vi "Version_2.0_Single_Column_Code.vi"() -> ()   [LabVIEW 2020] (continued)
                                n7327 = call "ProcessCompletionWaiter (SubVI).vi"("VISA Refnum in"=w7772) -> ()  [unwired: 11 in]
                                n7328 = local write "Start the Process"(FALSE ("Start the Process")) -> ()
                              }
                            }
                          }
                          frame #13 {
                            # "Clean the tubing with Sample"
                            n7329 = local read "N-S"() -> (w7774:i32)
                            n7330 = for {
                              N: w7774 -> [_]
                              n7331 = stacked-sequence {
                                frame #0 {
                                n7332 = local read "VISA Refnum in\nfor Pump"() -> (w7777:refnum<visa-resource-name>)
                                n7333 = local read "Port for \nSample"() -> (w7776:string)
                                n7334 = call "PortChanger (SubVI).vi"("Port Number"=w7776, "VISA Refnum in"=w7777) -> ()  [unwired: 10 in]
                                }
                                frame #1 {
                                n7335 = local read "VISA Refnum in\nfor Pump"() -> (w7778:refnum<visa-resource-name>)
                                n7336 = call "ProcessCompletionWaiter (SubVI).vi"("VISA Refnum in"=w7778) -> ()  [unwired: 11 in]
                                }
                                frame #2 {
                                n7337 = local read "VISA Refnum in\nfor Pump"() -> (w7783:refnum<visa-resource-name>)
                                n7338 = local read "Sample PickUp \nFlow Rate (ul/min)"() -> (w7780:dbl)
                                n7339 = local read "V-S"() -> (w7779:dbl)
                                n7340 = local read "Volume of Syringe"() -> (w7781:dbl)
                                n7341 = call "RPickUp(SubVI).vi"("Volume to be picked up"=w7779, "Volume of Syringe"=w7781, "Resolution of PickUP"=T2."Standard Pumping", "PickUp Flow Rate (ul/min)"=w7780, "VISA Refnum in"=w7783) -> ()  [unwired: 6 in, 1 out]
                                }
                                frame #3 {
                                n7342 = local read "Stopper that ends \nthe main loops"() -> (w7784:bool)
                                n7343 = local read "VISA Refnum in\nfor Pump"() -> (w7785:refnum<visa-resource-name>)
                                n7344 = case shown="True" w7784 {
                                frame False {
                                }
                                frame True {
                                n7345 = local read "VISA Refnum in\nfor Pump"() -> (w7786:refnum<visa-resource-name>)
                                n7346 = call "HardStopCurrentProcess (SubVI).vi"("VISA Refnum in"=w7786) -> ()  [unwired: 11 in]
                                }
                                }
                                n7347 = call "ProcessCompletionWaiter (SubVI).vi"("VISA Refnum in"=w7785) -> ()  [unwired: 11 in]
                                }
                                frame #4 {
                                n7348 = local read "VISA Refnum in\nfor Pump"() -> (w7788:refnum<visa-resource-name>)
                                n7349 = call "PortChanger (SubVI).vi"("Port Number"="1", "VISA Refnum in"=w7788) -> ()  [unwired: 10 in]
                                }
                                frame #5 {
                                n7350 = local read "Stopper that ends \nthe main loops"() -> (w7789:bool)
                                n7351 = local read "VISA Refnum in\nfor Pump"() -> (w7790:refnum<visa-resource-name>)
                                n7352 = case shown="True" w7789 {
                                frame False {
                                }
                                frame True {
                                n7353 = local read "VISA Refnum in\nfor Pump"() -> (w7791:refnum<visa-resource-name>)
                                n7354 = call "HardStopCurrentProcess (SubVI).vi"("VISA Refnum in"=w7791) -> ()  [unwired: 11 in]
                                }
                                }
                                n7355 = call "ProcessCompletionWaiter (SubVI).vi"("VISA Refnum in"=w7790) -> ()  [unwired: 11 in]
                                }
                                frame #6 {
                                n7356 = local read "VISA Refnum in\nfor Pump"() -> (w7796:refnum<visa-resource-name>)
                                n7357 = local read "Volume of Syringe"() -> (w7793:dbl)
                                n7358 = call "GoToAbsolutePosition(SubVI).vi"("Absolute Volume Position in Syringe (in ul)"=0.0 ("Volume to be picked up"), "Volume of Syringe"=w7793, "Resolution of Pumping"=T2."Standard Pumping" ("Resolution of PickUP"), "Flow Rate (ul/min)"=150.0 ("PickUp Flow Rate (ul/min)"), "VISA Refnum in"=w7796) -> ()  [unwired: 6 in, 1 out]
                                }
                                frame #7 {
                                n7359 = local read "Stopper that ends \nthe main loops"() -> (w7797:bool)
                                n7360 = local read "VISA Refnum in\nfor Pump"() -> (w7798:refnum<visa-resource-name>)
                                n7361 = case shown="True" w7797 {
                                frame False {
                                }
                                frame True {
                                n7362 = local read "VISA Refnum in\nfor Pump"() -> (w7799:refnum<visa-resource-name>)
                                n7363 = call "HardStopCurrentProcess (SubVI).vi"("VISA Refnum in"=w7799) -> ()  [unwired: 11 in]
                                }
                                }
                                n7364 = call "ProcessCompletionWaiter (SubVI).vi"("VISA Refnum in"=w7798) -> ()  [unwired: 11 in]
                                }
                              }
                              n7365 = local write "Pause Data Collection"(TRUE ("Pause Data Collection")) -> ()
                            }
                          }
                        }
                      }
                      frame #1 {
                        # "Pump Sample into Column-1"
                        n7366 = stacked-sequence {
                          frame #0 {
                            # "Switch to Port-3"
                            # "Port-3 of pump is connected to Sample"
                            n7367 = local read "VISA Refnum in\nfor Pump"() -> (w7804:refnum<visa-resource-name>)
                            n7368 = local read "Port for \nSample"() -> (w7803:string)
                            n7369 = call "PortChanger (SubVI).vi"("Port Number"=w7803, "VISA Refnum in"=w7804) -> ()  [unwired: 10 in]
                          }
                          frame #1 {
                            n7370 = local read "VISA Refnum in\nfor Pump"() -> (w7805:refnum<visa-resource-name>)
                            n7371 = call "ProcessCompletionWaiter (SubVI).vi"("VISA Refnum in"=w7805) -> ()  [unwired: 11 in]
                          }
                          frame #2 {
                            n7372 = local write "Valve V1 Open"(TRUE ("Valve V1 Open")) -> ()
                            n7373 = local write "Valve V2 Open"(FALSE ("Valve V2 Open")) -> ()
                            n7374 = local write "External Valve \nOpen"(FALSE ("External Valve \nOpen")) -> ()
                          }
                          frame #3 {
                            n7375 = local read "Apparent Volume\nof Syringe"() -> (w7809:dbl)
                            n7376 = local read "Sample Volume \nto be Pumped"() -> (w7812:dbl)
                            n7377 = Quotient & Remainder(x=w7812, y=w7809) -> (x-y*floor(x/y)=w7810:dbl, floor(x/y)=w7811:dbl)
                            n7378 = for {
                              N: w7811 -> [_]
                              n7379 = stacked-sequence {
                                frame #0 {
                                n7380 = local read "Sample PickUp \nFlow Rate (ul/min)"() -> (w7815:dbl)
                                n7381 = local read "Sample Pumping\nResolution"() -> (w7814:T2)
                                n7382 = local read "VISA Refnum in\nfor Pump"() -> (w7817:refnum<visa-resource-name>)
                                n7383 = local read "Apparent Volume\nof Syringe"() -> (w7813:dbl)
                                n7384 = local read "Volume of Syringe"() -> (w7816:dbl)
                                n7385 = call "RPickUp(SubVI).vi"("Volume to be picked up"=w7813, "Volume of Syringe"=w7816, "Resolution of PickUP"=w7814, "PickUp Flow Rate (ul/min)"=w7815, "VISA Refnum in"=w7817) -> ()  [unwired: 6 in, 1 out]
                                }
                                frame #1 {
                                n7386 = local read "Stopper that ends \nthe main loops"() -> (w7818:bool)
                                n7387 = local read "VISA Refnum in\nfor Pump"() -> (w7819:refnum<visa-resource-name>)
                                n7388 = case shown="True" w7818 {
                                frame False {
                                }
                                frame True {
                                n7389 = local read "VISA Refnum in\nfor Pump"() -> (w7820:refnum<visa-resource-name>)
                                n7390 = call "HardStopCurrentProcess (SubVI).vi"("VISA Refnum in"=w7820) -> ()  [unwired: 11 in]
                                }
                                }
                                n7391 = call "ProcessCompletionWaiter (SubVI).vi"("VISA Refnum in"=w7819) -> ()  [unwired: 11 in]
                                }
                                frame #2 {
                                # "Reads the initial Plunger Position for computing the volume dispensed"
                                n7392 = local read "VISA Refnum in\nfor Pump"() -> (w7822:refnum<visa-resource-name>)
                                n7393 = call "AbsolutePlungerPosition (SubVI).vi"("VISA Refnum in"=w7822) -> ("Plunger Position"=w7821:i32)  [unwired: 10 in]
                                n7394 = local write "Initial Plunger Position"(w7821) -> ()
                                }
                                frame #3 {
                                # "Switch to Port-2"
                                # "Port-2 of the pump is conncted to column-1 of chip"
                                n7395 = local read "VISA Refnum in\nfor Pump"() -> (w7824:refnum<visa-resource-name>)
                                n7396 = call "PortChanger (SubVI).vi"("Port Number"="2", "VISA Refnum in"=w7824) -> ()  [unwired: 10 in]
                                }
                                frame #4 {
                                n7397 = local read "Stopper that ends \nthe main loops"() -> (w7825:bool)
                                n7398 = local read "VISA Refnum in\nfor Pump"() -> (w7826:refnum<visa-resource-name>)
                                n7399 = case shown="True" w7825 {
                                frame False {
                                }
                                frame True {
                                n7400 = local read "VISA Refnum in\nfor Pump"() -> (w7827:refnum<visa-resource-name>)
                                n7401 = call "HardStopCurrentProcess (SubVI).vi"("VISA Refnum in"=w7827) -> ()  [unwired: 11 in]
                                }
                                }
                                n7402 = call "ProcessCompletionWaiter (SubVI).vi"("VISA Refnum in"=w7826) -> ()  [unwired: 11 in]
                                }
                                frame #5 {
                                # "Keeps the AMF valve after column-1 open and valve after column-2 closed"
                                n7403 = local read "Sample Dispense\nFlow Rate (ul/min)"() -> (w7831:dbl)
                                n7404 = local read "Sample Pumping\nResolution"() -> (w7830:T2)
                                n7405 = local read "VISA Refnum in\nfor Pump"() -> (w7833:refnum<visa-resource-name>)
                                n7406 = local write "Pause Data Collection"(FALSE ("Pause Data Collection")) -> ()
                                n7407 = local read "Volume of Syringe"() -> (w7832:dbl)
                                n7408 = call "GoToAbsolutePosition(SubVI).vi"("Absolute Volume Position in Syringe (in ul)"=0.0 ("Volume to be Dispensed"), "Volume of Syringe"=w7832, "Resolution of Pumping"=w7830, "Flow Rate (ul/min)"=w7831, "VISA Refnum in"=w7833) -> ()  [unwired: 6 in, 1 out]
                                }
                                frame #6 {
                                n7409 = local read "Sample Pumping\nResolution"() -> (w7835:T2)
                                n7410 = local read "VISA Refnum in\nfor Pump"() -> (w7837:refnum<visa-resource-name>)
                                n7411 = local read "Initial Plunger Position"() -> (w7836:dbl)
                                n7412 = local read "Volume of Syringe"() -> (w7834:dbl)
                                n7413 = while {
                                tunnel: w7836 -> [w7844]
                                tunnel: w7837 -> [w7843]
                                tunnel: w7835 -> [w7842]
                                tunnel: w7834 -> [w7841]
                                stop <- w7839 stop-if-true
                                n7414 = stacked-sequence {
                                tunnel: w7844 -> [w7851 _]
                                tunnel: w7843 -> [w7850 w7871]
                                tunnel: w7842 -> [w7849 _]
                                tunnel: w7841 -> [w7848 _]
                                tunnel: [_ w7869] -> w7839
                                frame #0 {
                                n7415 = call "AbsolutePlungerPosition (SubVI).vi"("VISA Refnum in"=w7850) -> ("Plunger Position"=w7847:i32)  [unwired: 10 in]
                                n7416 = case shown="\"Standard Pumping\", Default" w7849 {
                                tunnel: w7851 -> [w7856 w7865]
                                tunnel: w7847 -> [w7857 w7864]
                                tunnel: [w7855 w7862] -> w7846
                                tunnel: w7848 -> [w7854 w7863]
                                frame "Standard Pumping", Default {
                                n7417 = Subtract(x=w7856, y=w7857) -> (x-y=w7853:dbl)
                                n7418 = Absolute Value(x=w7853) -> (abs(x)=w7852:dbl)
                                n7419 = Multiply(x=w7852, y=w7854) -> (x*y=w7859:dbl)
                                n7420 = Divide(x=w7859, y=3000.0) -> (x/y=w7855:dbl)
                                }
                                frame "High Resolution Pumping" {
                                n7421 = Subtract(x=w7865, y=w7864) -> (x-y=w7861:dbl)
                                n7422 = Absolute Value(x=w7861) -> (abs(x)=w7860:dbl)
                                n7423 = Multiply(x=w7860, y=w7863) -> (x*y=w7867:dbl)
                                n7424 = Divide(x=w7867, y=24000.0) -> (x/y=w7862:dbl)
                                }
                                }
                                n7425 = local write "Volume being Injected \nin this process"(w7846) -> ()
                                }
                                frame #1 {
                                n7426 = call "LSPOneStatus (SubVI).vi"("VISA Refnum in"=w7871) -> ("read buffer"=w7873:string)  [unwired: 10 in]
                                n7427 = call <vilib>:"Trim Whitespace.vi"("string"=w7873) -> ("trimmed string"=w7872:string)  [unwired: 1 in]
                                n7428 = local read "Stopper that ends \nthe main loops"() -> (w7868:bool)
                                n7429 = Equal?(x=w7872, y="/0`\u0003") -> (x = y?=w7870:bool)
                                n7430 = Or(x=w7870, y=w7868) -> (x .or. y?=w7869:bool)
                                }
                                }
                                n7431 = Wait (ms)(milliseconds to wait=u32 100) -> ()  [unwired: 1 out]
                                n7432 = local read "Stopper that ends \nthe main loops"() -> (w7838:bool)
                                n7433 = case shown="True" w7838 {
                                frame False {
                                }
                                frame True {
                                n7434 = local read "VISA Refnum in\nfor Pump"() -> (w7845:refnum<visa-resource-name>)
                                n7435 = call "HardStopCurrentProcess (SubVI).vi"("VISA Refnum in"=w7845) -> ()  [unwired: 11 in]
                                }
                                }
                                }
                                }
                                frame #7 {
                                # "Chnage the pump port back to Sample"
                                n7436 = local read "VISA Refnum in\nfor Pump"() -> (w7876:refnum<visa-resource-name>)
                                n7437 = local read "Port for \nSample"() -> (w7875:string)
                                n7438 = local write "Pause Data Collection"(TRUE ("Pause Data Collection")) -> ()
                                n7439 = Wait (ms)(milliseconds to wait=u32 500) -> ()  [unwired: 1 out]
                                n7440 = call "PortChanger (SubVI).vi"("Port Number"=w7875, "VISA Refnum in"=w7876) -> ()  [unwired: 10 in]
                                }
                                frame #8 {
                                n7441 = local read "VISA Refnum in\nfor Pump"() -> (w7879:refnum<visa-resource-name>)
                                n7442 = local write "Volume being Injected \nin this process"(0.0 ("Volume being Injected \nin this process")) -> ()
                                n7443 = call "ProcessCompletionWaiter (SubVI).vi"("VISA Refnum in"=w7879) -> ()  [unwired: 11 in]
                                }
                              }
                            }
                            n7444 = local write "Reminder of the \nVolume to be \nPumped"(w7810) -> ()
                          }
                          frame #4 {
                            n7445 = stacked-sequence {
                              frame #0 {
                                n7446 = local read "Sample PickUp \nFlow Rate (ul/min)"() -> (w7883:dbl)
                                n7447 = local read "Sample Pumping\nResolution"() -> (w7882:T2)
                                n7448 = local read "VISA Refnum in\nfor Pump"() -> (w7885:refnum<visa-resource-name>)
                                n7449 = local read "Reminder of the \nVolume to be \nPumped"() -> (w7881:dbl)
                                n7450 = local read "Volume of Syringe"() -> (w7884:dbl)
                                n7451 = call "RPickUp(SubVI).vi"("Volume to be picked up"=w7881, "Volume of Syringe"=w7884, "Resolution of PickUP"=w7882, "PickUp Flow Rate (ul/min)"=w7883, "VISA Refnum in"=w7885) -> ()  [unwired: 6 in, 1 out]
                              }
                              frame #1 {
                                n7452 = local read "Stopper that ends \nthe main loops"() -> (w7886:bool)
                                n7453 = local read "VISA Refnum in\nfor Pump"() -> (w7887:refnum<visa-resource-name>)
                                n7454 = case shown="True" w7886 {
                                frame False {
                                }
                                frame True {
                                n7455 = local read "VISA Refnum in\nfor Pump"() -> (w7888:refnum<visa-resource-name>)
                                n7456 = call "HardStopCurrentProcess (SubVI).vi"("VISA Refnum in"=w7888) -> ()  [unwired: 11 in]
                                }
                                }
                                n7457 = call "ProcessCompletionWaiter (SubVI).vi"("VISA Refnum in"=w7887) -> ()  [unwired: 11 in]
                              }
                              frame #2 {
                                # "Reads the initial Plunger Position for computing the volume dispensed"
                                n7458 = local read "VISA Refnum in\nfor Pump"() -> (w7890:refnum<visa-resource-name>)
                                n7459 = call "AbsolutePlungerPosition (SubVI).vi"("VISA Refnum in"=w7890) -> ("Plunger Position"=w7889:i32)  [unwired: 10 in]
                                n7460 = local write "Initial Plunger Position"(w7889) -> ()
                              }
                              frame #3 {
                                # "Switch to Port-2"
                                # "Port-2 of the pump is conncted to column-1 of chip"
                                n7461 = local read "VISA Refnum in\nfor Pump"() -> (w7892:refnum<visa-resource-name>)
                                n7462 = call "PortChanger (SubVI).vi"("Port Number"="2", "VISA Refnum in"=w7892) -> ()  [unwired: 10 in]
                              }
                              frame #4 {
                                n7463 = local read "Stopper that ends \nthe main loops"() -> (w7893:bool)
                                n7464 = local read "VISA Refnum in\nfor Pump"() -> (w7894:refnum<visa-resource-name>)
                                n7465 = case shown="True" w7893 {
                                frame False {
                                }
                                frame True {
                                n7466 = local read "VISA Refnum in\nfor Pump"() -> (w7895:refnum<visa-resource-name>)
                                n7467 = call "HardStopCurrentProcess (SubVI).vi"("VISA Refnum in"=w7895) -> ()  [unwired: 11 in]
                                }
                                }
                                n7468 = call "ProcessCompletionWaiter (SubVI).vi"("VISA Refnum in"=w7894) -> ()  [unwired: 11 in]
                              }
                              frame #5 {
                                # "Keeps the AMF valve after column-1 open and valve after column-2 closed"
                                n7469 = local read "Sample Dispense\nFlow Rate (ul/min)"() -> (w7899:dbl)
                                n7470 = local read "Sample Pumping\nResolution"() -> (w7898:T2)
                                n7471 = local read "VISA Refnum in\nfor Pump"() -> (w7901:refnum<visa-resource-name>)
                                n7472 = local write "Pause Data Collection"(FALSE ("Pause Data Collection")) -> ()
                                n7473 = local read "Volume of Syringe"() -> (w7900:dbl)
                                n7474 = call "GoToAbsolutePosition(SubVI).vi"("Absolute Volume Position in Syringe (in ul)"=0.0 ("Volume to be Dispensed"), "Volume of Syringe"=w7900, "Resolution of Pumping"=w7898, "Flow Rate (ul/min)"=w7899, "VISA Refnum in"=w7901) -> ()  [unwired: 6 in, 1 out]
                              }
                              frame #6 {
                                n7475 = local read "Sample Pumping\nResolution"() -> (w7903:T2)
                                n7476 = local read "VISA Refnum in\nfor Pump"() -> (w7905:refnum<visa-resource-name>)
                                n7477 = local read "Initial Plunger Position"() -> (w7904:dbl)
                                n7478 = local read "Volume of Syringe"() -> (w7902:dbl)
                                n7479 = while {
                                tunnel: w7904 -> [w7912]
                                tunnel: w7905 -> [w7911]
                                tunnel: w7903 -> [w7910]
                                tunnel: w7902 -> [w7909]
                                stop <- w7907 stop-if-true
                                n7480 = stacked-sequence {
                                tunnel: w7912 -> [w7919 _]
                                tunnel: w7911 -> [w7918 w7939]
                                tunnel: w7910 -> [w7917 _]
                                tunnel: w7909 -> [w7916 _]
                                tunnel: [_ w7937] -> w7907
                                frame #0 {
                                n7481 = call "AbsolutePlungerPosition (SubVI).vi"("VISA Refnum in"=w7918) -> ("Plunger Position"=w7915:i32)  [unwired: 10 in]
                                n7482 = case shown="\"Standard Pumping\", Default" w7917 {
                                tunnel: w7919 -> [w7924 w7933]
                                tunnel: w7915 -> [w7925 w7932]
                                tunnel: [w7923 w7930] -> w7914
                                tunnel: w7916 -> [w7922 w7931]
                                frame "Standard Pumping", Default {
                                n7483 = Subtract(x=w7924, y=w7925) -> (x-y=w7921:dbl)
                                n7484 = Absolute Value(x=w7921) -> (abs(x)=w7920:dbl)
                                n7485 = Multiply(x=w7920, y=w7922) -> (x*y=w7927:dbl)
                                n7486 = Divide(x=w7927, y=3000.0) -> (x/y=w7923:dbl)
                                }
                                frame "High Resolution Pumping" {
                                n7487 = Subtract(x=w7933, y=w7932) -> (x-y=w7929:dbl)
                                n7488 = Absolute Value(x=w7929) -> (abs(x)=w7928:dbl)
                                n7489 = Multiply(x=w7928, y=w7931) -> (x*y=w7935:dbl)
                                n7490 = Divide(x=w7935, y=24000.0) -> (x/y=w7930:dbl)
                                }
                                }
                                n7491 = local write "Volume being Injected \nin this process"(w7914) -> ()
                                }
                                frame #1 {
                                n7492 = call "LSPOneStatus (SubVI).vi"("VISA Refnum in"=w7939) -> ("read buffer"=w7941:string)  [unwired: 10 in]
                                n7493 = call <vilib>:"Trim Whitespace.vi"("string"=w7941) -> ("trimmed string"=w7940:string)  [unwired: 1 in]
                                n7494 = local read "Stopper that ends \nthe main loops"() -> (w7936:bool)
                                n7495 = Equal?(x=w7940, y="/0`\u0003") -> (x = y?=w7938:bool)
                                n7496 = Or(x=w7938, y=w7936) -> (x .or. y?=w7937:bool)
                                }
                                }
                                n7497 = Wait (ms)(milliseconds to wait=u32 100) -> ()  [unwired: 1 out]
                                n7498 = local read "Stopper that ends \nthe main loops"() -> (w7906:bool)
                                n7499 = case shown="True" w7906 {
                                frame False {
                                }
                                frame True {
                                n7500 = local read "VISA Refnum in\nfor Pump"() -> (w7913:refnum<visa-resource-name>)
                                n7501 = call "HardStopCurrentProcess (SubVI).vi"("VISA Refnum in"=w7913) -> ()  [unwired: 11 in]
                                }
                                }
                                }
                              }
                              frame #7 {
                                n7502 = local write "Pause Data Collection"(TRUE ("Pause Data Collection")) -> ()
                                n7503 = Wait (ms)(milliseconds to wait=u32 500) -> ()  [unwired: 1 out]
                              }
                              frame #8 {
                                n7504 = local write "Volume being Injected \nin this process"(0.0 ("Volume being Injected \nin this process")) -> ()
                              }
                            }
                          }
                        }
                        n7505 = local write "Equilibriating \nColumn-2"(FALSE ("Equilibriating \nColumn-2")) -> ()
                        n7506 = local write "Affinity On"(TRUE ("Affinity On")) -> ()
                        n7507 = local write "Sample pumping \ninto Column-1"(TRUE ("Sample pumping \ninto Column-1")) -> ()
                      }
                      frame #2 {
                        # "Wash Column-1 with Buffer-A2"
                        n7508 = local write "Sample pumping \ninto Column-1"(FALSE ("Sample pumping \ninto Column-1")) -> ()
                        n7509 = stacked-sequence {
                          frame #0 {
                            # "Switch to Port-4/6"
                            # "Port-4/6 of pump is connected to Buffer-A2"
                            n7510 = local read "VISA Refnum in\nfor Pump"() -> (w7949:refnum<visa-resource-name>)
                            n7511 = local read "Port for \nA2-Wash"() -> (w7948:string)
                            n7512 = call "PortChanger (SubVI).vi"("Port Number"=w7948, "VISA Refnum in"=w7949) -> ()  [unwired: 10 in]
                          }
                          frame #1 {
                            n7513 = local read "VISA Refnum in\nfor Pump"() -> (w7950:refnum<visa-resource-name>)
                            n7514 = call "ProcessCompletionWaiter (SubVI).vi"("VISA Refnum in"=w7950) -> ()  [unwired: 11 in]
                          }
                          frame #2 {
                            n7515 = local write "Valve V1 Open"(TRUE ("Valve V1 Open")) -> ()
                            n7516 = local write "Valve V2 Open"(FALSE ("Valve V2 Open")) -> ()
                            n7517 = local write "External Valve \nOpen"(FALSE ("Elution of Column-2")) -> ()
                          }
                          frame #3 {
                            n7518 = local read "Buffer-A2 Volume \nto be Pumped"() -> (w7957:dbl)
                            n7519 = local read "Apparent Volume\nof Syringe"() -> (w7954:dbl)
                            n7520 = Quotient & Remainder(x=w7957, y=w7954) -> (x-y*floor(x/y)=w7955:dbl, floor(x/y)=w7956:dbl)
                            n7521 = for {
                              N: w7956 -> [_]
                              n7522 = stacked-sequence {
                                frame #0 {
                                n7523 = local read "Buffer-A2 PickUp \nFlow Rate (ul/min)"() -> (w7960:dbl)
                                n7524 = local read "Buffer-A2 Pumping\nResolution"() -> (w7959:T2)
                                n7525 = local read "VISA Refnum in\nfor Pump"() -> (w7962:refnum<visa-resource-name>)
                                n7526 = local read "Apparent Volume\nof Syringe"() -> (w7958:dbl)
                                n7527 = local read "Volume of Syringe"() -> (w7961:dbl)
                                n7528 = call "RPickUp(SubVI).vi"("Volume to be picked up"=w7958, "Volume of Syringe"=w7961, "Resolution of PickUP"=w7959, "PickUp Flow Rate (ul/min)"=w7960, "VISA Refnum in"=w7962) -> ()  [unwired: 6 in, 1 out]
                                }
                                frame #1 {
                                n7529 = local read "Stopper that ends \nthe main loops"() -> (w7963:bool)
                                n7530 = local read "VISA Refnum in\nfor Pump"() -> (w7964:refnum<visa-resource-name>)
                                n7531 = case shown="True" w7963 {
                                frame False {
                                }
                                frame True {
                                n7532 = local read "VISA Refnum in\nfor Pump"() -> (w7965:refnum<visa-resource-name>)
                                n7533 = call "HardStopCurrentProcess (SubVI).vi"("VISA Refnum in"=w7965) -> ()  [unwired: 11 in]
                                }
                                }
                                n7534 = call "ProcessCompletionWaiter (SubVI).vi"("VISA Refnum in"=w7964) -> ()  [unwired: 11 in]
                                }
                                frame #2 {
                                # "Reads the initial Plunger Position for computing the volume dispensed"
                                n7535 = local read "VISA Refnum in\nfor Pump"() -> (w7967:refnum<visa-resource-name>)
                                n7536 = call "AbsolutePlungerPosition (SubVI).vi"("VISA Refnum in"=w7967) -> ("Plunger Position"=w7966:i32)  [unwired: 10 in]
                                n7537 = local write "Initial Plunger Position"(w7966) -> ()
                                }
                                frame #3 {
                                # "Switch to Port-2"
                                # "Port-2 of the pump is conncted to column-1 of chip"
                                n7538 = local read "VISA Refnum in\nfor Pump"() -> (w7969:refnum<visa-resource-name>)
                                n7539 = call "PortChanger (SubVI).vi"("Port Number"="2", "VISA Refnum in"=w7969) -> ()  [unwired: 10 in]
                                }
                                frame #4 {
                                n7540 = local read "Stopper that ends \nthe main loops"() -> (w7970:bool)
                                n7541 = local read "VISA Refnum in\nfor Pump"() -> (w7971:refnum<visa-resource-name>)
                                n7542 = case shown="True" w7970 {
                                frame False {
                                }
                                frame True {
                                n7543 = local read "VISA Refnum in\nfor Pump"() -> (w7972:refnum<visa-resource-name>)
                                n7544 = call "HardStopCurrentProcess (SubVI).vi"("VISA Refnum in"=w7972) -> ()  [unwired: 11 in]
                                }
                                }
                                n7545 = call "ProcessCompletionWaiter (SubVI).vi"("VISA Refnum in"=w7971) -> ()  [unwired: 11 in]
                                }
                                frame #5 {
                                # "Keeps the AMF valve after column-1 open and valve after column-2 closed"
                                n7546 = local read "Buffer-A2 Dispense\nFlow Rate (ul/min)"() -> (w7976:dbl)
                                n7547 = local read "Buffer-A2 Pumping\nResolution"() -> (w7975:T2)
                                n7548 = local read "VISA Refnum in\nfor Pump"() -> (w7978:refnum<visa-resource-name>)
                                n7549 = local write "Pause Data Collection"(FALSE ("Pause Data Collection")) -> ()
                                n7550 = local read "Volume of Syringe"() -> (w7977:dbl)
                                n7551 = call "GoToAbsolutePosition(SubVI).vi"("Absolute Volume Position in Syringe (in ul)"=0.0 ("Volume to be Dispensed"), "Volume of Syringe"=w7977, "Resolution of Pumping"=w7975, "Flow Rate (ul/min)"=w7976, "VISA Refnum in"=w7978) -> ()  [unwired: 6 in, 1 out]
                                }
                                frame #6 {
                                n7552 = local read "Buffer-A2 Pumping\nResolution"() -> (w7980:T2)
                                n7553 = local read "VISA Refnum in\nfor Pump"() -> (w7982:refnum<visa-resource-name>)
                                n7554 = local read "Initial Plunger Position"() -> (w7981:dbl)
                                n7555 = local read "Volume of Syringe"() -> (w7979:dbl)
                                n7556 = while {
                                tunnel: w7981 -> [w7989]
                                tunnel: w7982 -> [w7988]
                                tunnel: w7980 -> [w7987]
                                tunnel: w7979 -> [w7986]
                                stop <- w7984 stop-if-true
                                n7557 = stacked-sequence {
                                tunnel: w7989 -> [w7996 _]
                                tunnel: w7988 -> [w7995 w8016]
                                tunnel: w7987 -> [w7994 _]
                                tunnel: w7986 -> [w7993 _]
                                tunnel: [_ w8014] -> w7984
                                frame #0 {
                                n7558 = call "AbsolutePlungerPosition (SubVI).vi"("VISA Refnum in"=w7995) -> ("Plunger Position"=w7992:i32)  [unwired: 10 in]
                                n7559 = case shown="\"Standard Pumping\", Default" w7994 {
                                tunnel: w7996 -> [w8001 w8010]
                                tunnel: w7992 -> [w8002 w8009]
                                tunnel: [w8000 w8007] -> w7991
                                tunnel: w7993 -> [w7999 w8008]
                                frame "Standard Pumping", Default {
                                n7560 = Subtract(x=w8001, y=w8002) -> (x-y=w7998:dbl)
                                n7561 = Absolute Value(x=w7998) -> (abs(x)=w7997:dbl)
                                n7562 = Multiply(x=w7997, y=w7999) -> (x*y=w8004:dbl)
                                n7563 = Divide(x=w8004, y=3000.0) -> (x/y=w8000:dbl)
                                }
                                frame "High Resolution Pumping" {
                                n7564 = Subtract(x=w8010, y=w8009) -> (x-y=w8006:dbl)
                                n7565 = Absolute Value(x=w8006) -> (abs(x)=w8005:dbl)
                                n7566 = Multiply(x=w8005, y=w8008) -> (x*y=w8012:dbl)
                                n7567 = Divide(x=w8012, y=24000.0) -> (x/y=w8007:dbl)
                                }
                                }
                                n7568 = local write "Volume being Injected \nin this process"(w7991) -> ()
                                }
                                frame #1 {
                                n7569 = call "LSPOneStatus (SubVI).vi"("VISA Refnum in"=w8016) -> ("read buffer"=w8018:string)  [unwired: 10 in]
                                n7570 = call <vilib>:"Trim Whitespace.vi"("string"=w8018) -> ("trimmed string"=w8017:string)  [unwired: 1 in]
                                n7571 = local read "Stopper that ends \nthe main loops"() -> (w8013:bool)
                                n7572 = Equal?(x=w8017, y="/0`\u0003") -> (x = y?=w8015:bool)
                                n7573 = Or(x=w8015, y=w8013) -> (x .or. y?=w8014:bool)
                                }
                                }
                                n7574 = Wait (ms)(milliseconds to wait=u32 100) -> ()  [unwired: 1 out]
                                n7575 = local read "Stopper that ends \nthe main loops"() -> (w7983:bool)
                                n7576 = case shown="True" w7983 {
                                frame False {
                                }
                                frame True {
                                n7577 = local read "VISA Refnum in\nfor Pump"() -> (w7990:refnum<visa-resource-name>)
                                n7578 = call "HardStopCurrentProcess (SubVI).vi"("VISA Refnum in"=w7990) -> ()  [unwired: 11 in]
                                }
                                }
                                }
                                }
                                frame #7 {
                                # "Change the port back to Buffer-A2"
                                n7579 = local read "VISA Refnum in\nfor Pump"() -> (w8021:refnum<visa-resource-name>)
                                n7580 = local read "Port for \nA2-Wash"() -> (w8020:string)
                                n7581 = local write "Pause Data Collection"(TRUE ("Pause Data Collection")) -> ()
                                n7582 = Wait (ms)(milliseconds to wait=u32 500) -> ()  [unwired: 1 out]
                                n7583 = call "PortChanger (SubVI).vi"("Port Number"=w8020, "VISA Refnum in"=w8021) -> ()  [unwired: 10 in]
                                }
                                frame #8 {
                                n7584 = local read "VISA Refnum in\nfor Pump"() -> (w8024:refnum<visa-resource-name>)
                                n7585 = local write "Volume being Injected \nin this process"(0.0 ("Volume being Injected \nin this process")) -> ()
                                n7586 = call "ProcessCompletionWaiter (SubVI).vi"("VISA Refnum in"=w8024) -> ()  [unwired: 11 in]
                                }
                              }
                            }
                            n7587 = local write "Reminder of the \nVolume to be \nPumped"(w7955) -> ()
                          }
                          frame #4 {
                            n7588 = stacked-sequence {
                              frame #0 {
                                n7589 = local read "Buffer-A2 PickUp \nFlow Rate (ul/min)"() -> (w8028:dbl)
                                n7590 = local read "Buffer-A2 Pumping\nResolution"() -> (w8027:T2)
                                n7591 = local read "VISA Refnum in\nfor Pump"() -> (w8030:refnum<visa-resource-name>)
                                n7592 = local read "Reminder of the \nVolume to be \nPumped"() -> (w8026:dbl)
                                n7593 = local read "Volume of Syringe"() -> (w8029:dbl)
                                n7594 = call "RPickUp(SubVI).vi"("Volume to be picked up"=w8026, "Volume of Syringe"=w8029, "Resolution of PickUP"=w8027, "PickUp Flow Rate (ul/min)"=w8028, "VISA Refnum in"=w8030) -> ()  [unwired: 6 in, 1 out]
                              }
                              frame #1 {
                                n7595 = local read "Stopper that ends \nthe main loops"() -> (w8031:bool)
                                n7596 = local read "VISA Refnum in\nfor Pump"() -> (w8032:refnum<visa-resource-name>)
                                n7597 = case shown="True" w8031 {
                                frame False {
                                }
                                frame True {
                                n7598 = local read "VISA Refnum in\nfor Pump"() -> (w8033:refnum<visa-resource-name>)
                                n7599 = call "HardStopCurrentProcess (SubVI).vi"("VISA Refnum in"=w8033) -> ()  [unwired: 11 in]
                                }
                                }
                                n7600 = call "ProcessCompletionWaiter (SubVI).vi"("VISA Refnum in"=w8032) -> ()  [unwired: 11 in]
                              }
                              frame #2 {
                                # "Reads the initial Plunger Position for computing the volume dispensed"
                                n7601 = local read "VISA Refnum in\nfor Pump"() -> (w8035:refnum<visa-resource-name>)
                                n7602 = call "AbsolutePlungerPosition (SubVI).vi"("VISA Refnum in"=w8035) -> ("Plunger Position"=w8034:i32)  [unwired: 10 in]
                                n7603 = local write "Initial Plunger Position"(w8034) -> ()
                              }
                              frame #3 {
                                # "Switch to Port-2"
                                # "Port-2 of the pump is conncted to column-1 of chip"
                                n7604 = local read "VISA Refnum in\nfor Pump"() -> (w8037:refnum<visa-resource-name>)
                                n7605 = call "PortChanger (SubVI).vi"("Port Number"="2", "VISA Refnum in"=w8037) -> ()  [unwired: 10 in]
                              }
                              frame #4 {
                                n7606 = local read "Stopper that ends \nthe main loops"() -> (w8038:bool)
                                n7607 = local read "VISA Refnum in\nfor Pump"() -> (w8039:refnum<visa-resource-name>)
                                n7608 = case shown="True" w8038 {
                                frame False {
                                }
                                frame True {
                                n7609 = local read "VISA Refnum in\nfor Pump"() -> (w8040:refnum<visa-resource-name>)
                                n7610 = call "HardStopCurrentProcess (SubVI).vi"("VISA Refnum in"=w8040) -> ()  [unwired: 11 in]
                                }
                                }
                                n7611 = call "ProcessCompletionWaiter (SubVI).vi"("VISA Refnum in"=w8039) -> ()  [unwired: 11 in]
                              }
                              frame #5 {
                                # "Keeps the AMF valve after column-1 open and valve after column-2 closed"
                                n7612 = local read "Buffer-A2 Dispense\nFlow Rate (ul/min)"() -> (w8044:dbl)
                                n7613 = local read "Buffer-A2 Pumping\nResolution"() -> (w8043:T2)
                                n7614 = local read "VISA Refnum in\nfor Pump"() -> (w8046:refnum<visa-resource-name>)
                                n7615 = local write "Pause Data Collection"(FALSE ("Pause Data Collection")) -> ()
                                n7616 = local read "Volume of Syringe"() -> (w8045:dbl)
                                n7617 = call "GoToAbsolutePosition(SubVI).vi"("Absolute Volume Position in Syringe (in ul)"=0.0 ("Volume to be Dispensed"), "Volume of Syringe"=w8045, "Resolution of Pumping"=w8043, "Flow Rate (ul/min)"=w8044, "VISA Refnum in"=w8046) -> ()  [unwired: 6 in, 1 out]
                              }
                              frame #6 {
                                n7618 = local read "Buffer-A2 Pumping\nResolution"() -> (w8048:T2)
                                n7619 = local read "VISA Refnum in\nfor Pump"() -> (w8050:refnum<visa-resource-name>)
                                n7620 = local read "Initial Plunger Position"() -> (w8049:dbl)
                                n7621 = local read "Volume of Syringe"() -> (w8047:dbl)
                                n7622 = while {
                                tunnel: w8049 -> [w8057]
                                tunnel: w8050 -> [w8056]
                                tunnel: w8048 -> [w8055]
                                tunnel: w8047 -> [w8054]
                                stop <- w8052 stop-if-true
                                n7623 = stacked-sequence {
                                tunnel: w8057 -> [w8064 _]
                                tunnel: w8056 -> [w8063 w8084]
                                tunnel: w8055 -> [w8062 _]
                                tunnel: w8054 -> [w8061 _]
                                tunnel: [_ w8082] -> w8052
                                frame #0 {
                                n7624 = call "AbsolutePlungerPosition (SubVI).vi"("VISA Refnum in"=w8063) -> ("Plunger Position"=w8060:i32)  [unwired: 10 in]
                                n7625 = case shown="\"Standard Pumping\", Default" w8062 {
                                tunnel: w8064 -> [w8069 w8078]
                                tunnel: w8060 -> [w8070 w8077]
                                tunnel: [w8068 w8075] -> w8059
                                tunnel: w8061 -> [w8067 w8076]
                                frame "Standard Pumping", Default {
                                n7626 = Subtract(x=w8069, y=w8070) -> (x-y=w8066:dbl)
                                n7627 = Absolute Value(x=w8066) -> (abs(x)=w8065:dbl)
                                n7628 = Multiply(x=w8065, y=w8067) -> (x*y=w8072:dbl)
                                n7629 = Divide(x=w8072, y=3000.0) -> (x/y=w8068:dbl)
                                }
                                frame "High Resolution Pumping" {
                                n7630 = Subtract(x=w8078, y=w8077) -> (x-y=w8074:dbl)
                                n7631 = Absolute Value(x=w8074) -> (abs(x)=w8073:dbl)
                                n7632 = Multiply(x=w8073, y=w8076) -> (x*y=w8080:dbl)
                                n7633 = Divide(x=w8080, y=24000.0) -> (x/y=w8075:dbl)
                                }
                                }
                                n7634 = local write "Volume being Injected \nin this process"(w8059) -> ()
                                }
                                frame #1 {
                                n7635 = call "LSPOneStatus (SubVI).vi"("VISA Refnum in"=w8084) -> ("read buffer"=w8086:string)  [unwired: 10 in]
                                n7636 = call <vilib>:"Trim Whitespace.vi"("string"=w8086) -> ("trimmed string"=w8085:string)  [unwired: 1 in]
                                n7637 = local read "Stopper that ends \nthe main loops"() -> (w8081:bool)
                                n7638 = Equal?(x=w8085, y="/0`\u0003") -> (x = y?=w8083:bool)
                                n7639 = Or(x=w8083, y=w8081) -> (x .or. y?=w8082:bool)
                                }
                                }
                                n7640 = Wait (ms)(milliseconds to wait=u32 100) -> ()  [unwired: 1 out]
                                n7641 = local read "Stopper that ends \nthe main loops"() -> (w8051:bool)
                                n7642 = case shown="True" w8051 {
                                frame False {
                                }
                                frame True {
                                n7643 = local read "VISA Refnum in\nfor Pump"() -> (w8058:refnum<visa-resource-name>)
                                n7644 = call "HardStopCurrentProcess (SubVI).vi"("VISA Refnum in"=w8058) -> ()  [unwired: 11 in]
                                }
                                }
                                }
                              }
                              frame #7 {
                                n7645 = local write "Pause Data Collection"(TRUE ("Pause Data Collection")) -> ()
                                n7646 = Wait (ms)(milliseconds to wait=u32 500) -> ()  [unwired: 1 out]
                              }
                              frame #8 {
                                n7647 = local write "Volume being Injected \nin this process"(0.0 ("Volume being Injected \nin this process")) -> ()
                                n7648 = local write "Start the Process"(FALSE ("Start the Process")) -> ()
                              }
                            }
                          }
                        }
                        n7649 = local write "Washing Column-1"(TRUE ("Washing Column-1")) -> ()
                      }
                      frame #3 {
                        # "Elute Column-1 with Buffer-B"
                        n7650 = stacked-sequence {
                          frame #0 {
                            # "Switch to Port-4/6"
                            # "Port-4/6 of pump is connected to Buffer-A2"
                            n7651 = local read "VISA Refnum in\nfor Pump"() -> (w8096:refnum<visa-resource-name>)
                            n7652 = local read "Port for \nB-Elution"() -> (w8095:string)
                            n7653 = call "PortChanger (SubVI).vi"("Port Number"=w8095, "VISA Refnum in"=w8096) -> ()  [unwired: 10 in]
                          }
                          frame #1 {
                            n7654 = local read "VISA Refnum in\nfor Pump"() -> (w8097:refnum<visa-resource-name>)
                            n7655 = call "ProcessCompletionWaiter (SubVI).vi"("VISA Refnum in"=w8097) -> ()  [unwired: 11 in]
                          }
                          frame #2 {
                            n7656 = local write "Valve V1 Open"(TRUE ("Valve V1 Open")) -> ()
                            n7657 = local write "Valve V2 Open"(FALSE ("Valve V2 Open")) -> ()
                            n7658 = local write "External Valve \nOpen"(FALSE ("Elution of Column-2")) -> ()
                          }
                          frame #3 {
                            n7659 = local read "Buffer-B Volume \nto be  Pumped"() -> (w8104:dbl)
                            n7660 = local read "Apparent Volume\nof Syringe"() -> (w8101:dbl)
                            n7661 = Quotient & Remainder(x=w8104, y=w8101) -> (x-y*floor(x/y)=w8102:dbl, floor(x/y)=w8103:dbl)
                            n7662 = for {
                              N: w8103 -> [_]
                              n7663 = stacked-sequence {
                                frame #0 {
                                n7664 = local read "Buffer-B PickUp \nFlow Rate (ul/min)"() -> (w8107:dbl)
                                n7665 = local read "Buffer-B Pumping\nResolution"() -> (w8106:T2)
                                n7666 = local read "VISA Refnum in\nfor Pump"() -> (w8109:refnum<visa-resource-name>)
                                n7667 = local read "Apparent Volume\nof Syringe"() -> (w8105:dbl)
                                n7668 = local read "Volume of Syringe"() -> (w8108:dbl)
                                n7669 = call "RPickUp(SubVI).vi"("Volume to be picked up"=w8105, "Volume of Syringe"=w8108, "Resolution of PickUP"=w8106, "PickUp Flow Rate (ul/min)"=w8107, "VISA Refnum in"=w8109) -> ()  [unwired: 6 in, 1 out]
                                }
                                frame #1 {
                                n7670 = local read "Stopper that ends \nthe main loops"() -> (w8110:bool)
                                n7671 = local read "VISA Refnum in\nfor Pump"() -> (w8111:refnum<visa-resource-name>)
                                n7672 = case shown="True" w8110 {
                                frame False {
                                }
                                frame True {
                                n7673 = local read "VISA Refnum in\nfor Pump"() -> (w8112:refnum<visa-resource-name>)
                                n7674 = call "HardStopCurrentProcess (SubVI).vi"("VISA Refnum in"=w8112) -> ()  [unwired: 11 in]
                                }
                                }
                                n7675 = call "ProcessCompletionWaiter (SubVI).vi"("VISA Refnum in"=w8111) -> ()  [unwired: 11 in]
                                }
                                frame #2 {
                                # "Reads the initial Plunger Position for computing the volume dispensed"
                                n7676 = local read "VISA Refnum in\nfor Pump"() -> (w8114:refnum<visa-resource-name>)
                                n7677 = call "AbsolutePlungerPosition (SubVI).vi"("VISA Refnum in"=w8114) -> ("Plunger Position"=w8113:i32)  [unwired: 10 in]
                                n7678 = local write "Initial Plunger Position"(w8113) -> ()
                                }
                                frame #3 {
                                # "Switch to Port-2"
                                # "Port-2 of the pump is conncted to column-1 of chip"
                                n7679 = local read "VISA Refnum in\nfor Pump"() -> (w8116:refnum<visa-resource-name>)
                                n7680 = call "PortChanger (SubVI).vi"("Port Number"="8", "VISA Refnum in"=w8116) -> ()  [unwired: 10 in]
                                }
                                frame #4 {
                                n7681 = local read "Stopper that ends \nthe main loops"() -> (w8117:bool)
                                n7682 = local read "VISA Refnum in\nfor Pump"() -> (w8118:refnum<visa-resource-name>)
                                n7683 = case shown="True" w8117 {
                                frame False {
                                }
                                frame True {
                                n7684 = local read "VISA Refnum in\nfor Pump"() -> (w8119:refnum<visa-resource-name>)
                                n7685 = call "HardStopCurrentProcess (SubVI).vi"("VISA Refnum in"=w8119) -> ()  [unwired: 11 in]
                                }
                                }
                                n7686 = call "ProcessCompletionWaiter (SubVI).vi"("VISA Refnum in"=w8118) -> ()  [unwired: 11 in]
                                }
                                frame #5 {
                                # "Keeps the AMF valve after column-1 open and valve after column-2 closed"
                                n7687 = local read "Buffer-B Dispense\nFlow Rate (ul/min)"() -> (w8123:dbl)
                                n7688 = local read "Buffer-B Pumping\nResolution"() -> (w8122:T2)
                                n7689 = local read "VISA Refnum in\nfor Pump"() -> (w8125:refnum<visa-resource-name>)
                                n7690 = local write "Pause Data Collection"(FALSE ("Pause Data Collection")) -> ()
                                n7691 = local read "Volume of Syringe"() -> (w8124:dbl)
                                n7692 = call "GoToAbsolutePosition(SubVI).vi"("Absolute Volume Position in Syringe (in ul)"=0.0 ("Volume to be Dispensed"), "Volume of Syringe"=w8124, "Resolution of Pumping"=w8122, "Flow Rate (ul/min)"=w8123, "VISA Refnum in"=w8125) -> ()  [unwired: 6 in, 1 out]
                                }
                                frame #6 {
                                n7693 = local read "Buffer-B Pumping\nResolution"() -> (w8127:T2)
                                n7694 = local read "VISA Refnum in\nfor Pump"() -> (w8129:refnum<visa-resource-name>)
                                n7695 = local read "Initial Plunger Position"() -> (w8128:dbl)
                                n7696 = local read "Volume of Syringe"() -> (w8126:dbl)
                                n7697 = while {
                                tunnel: w8128 -> [w8136]
                                tunnel: w8129 -> [w8135]
                                tunnel: w8127 -> [w8134]
                                tunnel: w8126 -> [w8133]
                                stop <- w8131 stop-if-true
                                n7698 = stacked-sequence {
                                tunnel: w8136 -> [w8143 _]
                                tunnel: w8135 -> [w8142 w8163]
                                tunnel: w8134 -> [w8141 _]
                                tunnel: w8133 -> [w8140 _]
                                tunnel: [_ w8161] -> w8131
                                frame #0 {
                                n7699 = call "AbsolutePlungerPosition (SubVI).vi"("VISA Refnum in"=w8142) -> ("Plunger Position"=w8139:i32)  [unwired: 10 in]
                                n7700 = case shown="\"Standard Pumping\", Default" w8141 {
                                tunnel: w8143 -> [w8148 w8157]
                                tunnel: w8139 -> [w8149 w8156]
                                tunnel: [w8147 w8154] -> w8138
                                tunnel: w8140 -> [w8146 w8155]
                                frame "Standard Pumping", Default {
                                n7701 = Subtract(x=w8148, y=w8149) -> (x-y=w8145:dbl)
                                n7702 = Absolute Value(x=w8145) -> (abs(x)=w8144:dbl)
                                n7703 = Multiply(x=w8144, y=w8146) -> (x*y=w8151:dbl)
                                n7704 = Divide(x=w8151, y=3000.0) -> (x/y=w8147:dbl)
                                }
                                frame "High Resolution Pumping" {
                                n7705 = Subtract(x=w8157, y=w8156) -> (x-y=w8153:dbl)
                                n7706 = Absolute Value(x=w8153) -> (abs(x)=w8152:dbl)
                                n7707 = Multiply(x=w8152, y=w8155) -> (x*y=w8159:dbl)
                                n7708 = Divide(x=w8159, y=24000.0) -> (x/y=w8154:dbl)
                                }
                                }
                                n7709 = local write "Volume being Injected \nin this process"(w8138) -> ()
                                }
                                frame #1 {
                                n7710 = call "LSPOneStatus (SubVI).vi"("VISA Refnum in"=w8163) -> ("read buffer"=w8165:string)  [unwired: 10 in]
                                n7711 = call <vilib>:"Trim Whitespace.vi"("string"=w8165) -> ("trimmed string"=w8164:string)  [unwired: 1 in]
                                n7712 = local read "Stopper that ends \nthe main loops"() -> (w8160:bool)
                                n7713 = Equal?(x=w8164, y="/0`\u0003") -> (x = y?=w8162:bool)
                                n7714 = Or(x=w8162, y=w8160) -> (x .or. y?=w8161:bool)
                                }
                                }
                                n7715 = Wait (ms)(milliseconds to wait=u32 100) -> ()  [unwired: 1 out]
                                n7716 = local read "Stopper that ends \nthe main loops"() -> (w8130:bool)
                                n7717 = case shown="True" w8130 {
                                frame False {
                                }
                                frame True {
                                n7718 = local read "VISA Refnum in\nfor Pump"() -> (w8137:refnum<visa-resource-name>)
                                n7719 = call "HardStopCurrentProcess (SubVI).vi"("VISA Refnum in"=w8137) -> ()  [unwired: 11 in]
                                }
                                }
                                }
                                }
                                frame #7 {
                                # "Change the port back to Buffer-A2"
                                n7720 = local read "VISA Refnum in\nfor Pump"() -> (w8168:refnum<visa-resource-name>)
                                n7721 = local read "Port for \nB-Elution"() -> (w8167:string)
                                n7722 = local write "Pause Data Collection"(TRUE ("Pause Data Collection")) -> ()
                                n7723 = Wait (ms)(milliseconds to wait=u32 500) -> ()  [unwired: 1 out]
                                n7724 = call "PortChanger (SubVI).vi"("Port Number"=w8167, "VISA Refnum in"=w8168) -> ()  [unwired: 10 in]
                                }
                                frame #8 {
                                n7725 = local read "VISA Refnum in\nfor Pump"() -> (w8171:refnum<visa-resource-name>)
                                n7726 = local write "Volume being Injected \nin this process"(0.0 ("Volume being Injected \nin this process")) -> ()
                                n7727 = call "ProcessCompletionWaiter (SubVI).vi"("VISA Refnum in"=w8171) -> ()  [unwired: 11 in]
                                }
                              }
                            }
                            n7728 = local write "Reminder of the \nVolume to be \nPumped"(w8102) -> ()
                          }
                          frame #4 {
                            n7729 = stacked-sequence {
                              frame #0 {
                                n7730 = local read "Buffer-B PickUp \nFlow Rate (ul/min)"() -> (w8175:dbl)
                                n7731 = local read "Buffer-B Pumping\nResolution"() -> (w8174:T2)
                                n7732 = local read "VISA Refnum in\nfor Pump"() -> (w8177:refnum<visa-resource-name>)
                                n7733 = local read "Reminder of the \nVolume to be \nPumped"() -> (w8173:dbl)
                                n7734 = local read "Volume of Syringe"() -> (w8176:dbl)
                                n7735 = call "RPickUp(SubVI).vi"("Volume to be picked up"=w8173, "Volume of Syringe"=w8176, "Resolution of PickUP"=w8174, "PickUp Flow Rate (ul/min)"=w8175, "VISA Refnum in"=w8177) -> ()  [unwired: 6 in, 1 out]
                              }
                              frame #1 {
                                n7736 = local read "Stopper that ends \nthe main loops"() -> (w8178:bool)
                                n7737 = local read "VISA Refnum in\nfor Pump"() -> (w8179:refnum<visa-resource-name>)
                                n7738 = case shown="True" w8178 {
                                frame False {
                                }
                                frame True {
                                n7739 = local read "VISA Refnum in\nfor Pump"() -> (w8180:refnum<visa-resource-name>)
                                n7740 = call "HardStopCurrentProcess (SubVI).vi"("VISA Refnum in"=w8180) -> ()  [unwired: 11 in]
                                }
                                }
                                n7741 = call "ProcessCompletionWaiter (SubVI).vi"("VISA Refnum in"=w8179) -> ()  [unwired: 11 in]
                              }
                              frame #2 {
                                # "Reads the initial Plunger Position for computing the volume dispensed"
                                n7742 = local read "VISA Refnum in\nfor Pump"() -> (w8182:refnum<visa-resource-name>)
                                n7743 = call "AbsolutePlungerPosition (SubVI).vi"("VISA Refnum in"=w8182) -> ("Plunger Position"=w8181:i32)  [unwired: 10 in]
                                n7744 = local write "Initial Plunger Position"(w8181) -> ()
                              }
                              frame #3 {
                                # "Switch to Port-2"
                                # "Port-2 of the pump is conncted to column-1 of chip"
                                n7745 = local read "VISA Refnum in\nfor Pump"() -> (w8184:refnum<visa-resource-name>)
                                n7746 = call "PortChanger (SubVI).vi"("Port Number"="8", "VISA Refnum in"=w8184) -> ()  [unwired: 10 in]
                              }
                              frame #4 {
                                n7747 = local read "Stopper that ends \nthe main loops"() -> (w8185:bool)
                                n7748 = local read "VISA Refnum in\nfor Pump"() -> (w8186:refnum<visa-resource-name>)
                                n7749 = case shown="True" w8185 {
                                frame False {
                                }
                                frame True {
                                n7750 = local read "VISA Refnum in\nfor Pump"() -> (w8187:refnum<visa-resource-name>)
                                n7751 = call "HardStopCurrentProcess (SubVI).vi"("VISA Refnum in"=w8187) -> ()  [unwired: 11 in]
                                }
                                }
                                n7752 = call "ProcessCompletionWaiter (SubVI).vi"("VISA Refnum in"=w8186) -> ()  [unwired: 11 in]
                              }
                              frame #5 {
                                # "Keeps the AMF valve after column-1 open and valve after column-2 closed"
                                n7753 = local read "Buffer-B Dispense\nFlow Rate (ul/min)"() -> (w8191:dbl)
                                n7754 = local read "Buffer-B Pumping\nResolution"() -> (w8190:T2)
                                n7755 = local read "VISA Refnum in\nfor Pump"() -> (w8193:refnum<visa-resource-name>)
                                n7756 = local write "Pause Data Collection"(FALSE ("Pause Data Collection")) -> ()
                                n7757 = local read "Volume of Syringe"() -> (w8192:dbl)
                                n7758 = call "GoToAbsolutePosition(SubVI).vi"("Absolute Volume Position in Syringe (in ul)"=0.0 ("Volume to be Dispensed"), "Volume of Syringe"=w8192, "Resolution of Pumping"=w8190, "Flow Rate (ul/min)"=w8191, "VISA Refnum in"=w8193) -> ()  [unwired: 6 in, 1 out]
                              }
                              frame #6 {
                                n7759 = local read "Buffer-B Pumping\nResolution"() -> (w8195:T2)
                                n7760 = local read "VISA Refnum in\nfor Pump"() -> (w8197:refnum<visa-resource-name>)
                                n7761 = local read "Initial Plunger Position"() -> (w8196:dbl)
                                n7762 = local read "Volume of Syringe"() -> (w8194:dbl)
                                n7763 = while {
                                tunnel: w8196 -> [w8204]
                                tunnel: w8197 -> [w8203]
                                tunnel: w8195 -> [w8202]
                                tunnel: w8194 -> [w8201]
                                stop <- w8199 stop-if-true
                                n7764 = stacked-sequence {
                                tunnel: w8204 -> [w8211 _]
                                tunnel: w8203 -> [w8210 w8233]
                                tunnel: w8202 -> [w8209 _]
                                tunnel: w8201 -> [w8208 _]
                                tunnel: [_ w8231] -> w8199
                                frame #0 {
                                n7765 = call "AbsolutePlungerPosition (SubVI).vi"("VISA Refnum in"=w8210) -> ("Plunger Position"=w8207:i32)  [unwired: 10 in]
                                n7766 = case shown="\"Standard Pumping\", Default" w8209 {
                                tunnel: w8211 -> [w8216 w8225]
                                tunnel: w8207 -> [w8217 w8224]
                                tunnel: [w8215 w8222] -> w8206
                                tunnel: w8208 -> [w8214 w8223]
                                frame "Standard Pumping", Default {
                                n7767 = Subtract(x=w8216, y=w8217) -> (x-y=w8213:dbl)
                                n7768 = Absolute Value(x=w8213) -> (abs(x)=w8212:dbl)
                                n7769 = Multiply(x=w8212, y=w8214) -> (x*y=w8219:dbl)
                                n7770 = Divide(x=w8219, y=3000.0) -> (x/y=w8215:dbl)
                                }
                                frame "High Resolution Pumping" {
                                n7771 = Subtract(x=w8225, y=w8224) -> (x-y=w8221:dbl)
                                n7772 = Absolute Value(x=w8221) -> (abs(x)=w8220:dbl)
                                n7773 = Multiply(x=w8220, y=w8223) -> (x*y=w8227:dbl)
                                n7774 = Divide(x=w8227, y=24000.0) -> (x/y=w8222:dbl)
                                }
                                }
                                n7775 = local write "Volume being Injected \nin this process"(w8206) -> ()
                                }
                                frame #1 {
                                n7776 = call "LSPOneStatus (SubVI).vi"("VISA Refnum in"=w8233) -> ("read buffer"=w8235:string)  [unwired: 10 in]
                                n7777 = call <vilib>:"Trim Whitespace.vi"("string"=w8235) -> ("trimmed string"=w8234:string)  [unwired: 1 in]
                                n7778 = local read "Stopper that ends \nthe main loops"() -> (w8229:bool)
                                n7779 = Equal?(x=w8234, y="/0`\u0003") -> (x = y?=w8232:bool)
                                n7780 = local read "Divert Sample \nonto Grid"() -> (w8230:bool)
                                n7781 = Or(x=w8229, y=w8230) -> (x .or. y?=w8228:bool)
                                n7782 = Or(x=w8232, y=w8228) -> (x .or. y?=w8231:bool)
                                }
                                }
                                n7783 = Wait (ms)(milliseconds to wait=u32 100) -> ()  [unwired: 1 out]
                                n7784 = local read "Stopper that ends \nthe main loops"() -> (w8198:bool)
                                n7785 = case shown="True" w8198 {
                                frame False {
                                }
                                frame True {
                                n7786 = local read "VISA Refnum in\nfor Pump"() -> (w8205:refnum<visa-resource-name>)
                                n7787 = call "HardStopCurrentProcess (SubVI).vi"("VISA Refnum in"=w8205) -> ()  [unwired: 11 in]
                                }
                                }
                                }
                              }
                              frame #7 {
                                n7788 = local read "Volume being Injected \nin this process"() -> (w8239:dbl)
                                n7789 = local read "VISA Refnum in\nfor Pump"() -> (w8241:refnum<visa-resource-name>)
                                n7790 = call "AbsolutePlungerPosition (SubVI).vi"("VISA Refnum in"=w8241) -> ("Plunger Position"=w8240:i32)  [unwired: 10 in]
                                n7791 = local write "Pause Data Collection"(TRUE) -> ()
                                n7792 = local write "True Volume being \ninjected in this\nprocess"(w8239) -> ()
                                n7793 = local write "Position\nNow"(w8240) -> ()
                                n7794 = Wait (ms)(milliseconds to wait=u32 500) -> ()  [unwired: 1 out]
                              }
                              frame #8 {
                                # "Sample Deposition onto EM-Grid"
                                n7795 = local read "Divert Sample \nonto Grid"() -> (w8242:bool)
                                n7796 = case shown="True" w8242 {
                                frame False {
                                }
                                frame True {
                                n7797 = stacked-sequence {
                                frame #0 {
                                # "Discard the initial volume of fluid that is present in the channel prior to detection"
                                n7798 = local read "Buffer-C2 Pumping\nResolution"() -> (w8250:T2)
                                n7799 = local read "Initial Plunger Position"() -> (w8249:dbl)
                                n7800 = local read "VISA Refnum in\nfor Pump"() -> (w8251:refnum<visa-resource-name>)
                                n7801 = local read "Position\nNow"() -> (w8247:dbl)
                                n7802 = local read "Volume of Syringe"() -> (w8248:dbl)
                                n7803 = local write "Pause Data Collection"(FALSE) -> ()
                                n7804 = while {
                                tunnel: w8251 -> [w8260]
                                tunnel: w8250 -> [w8259]
                                tunnel: w8249 -> [w8255]
                                tunnel: w8248 -> [w8258]
                                tunnel: w8247 -> [w8254]
                                stop <- w8256 stop-if-true
                                n7805 = stacked-sequence {
                                tunnel: w8260 -> [w8266 w8288 w8320]
                                tunnel: w8259 -> [w8265 w8287 _]
                                tunnel: w8255 -> [w8263 _ _]
                                tunnel: w8258 -> [w8262 w8285 _]
                                tunnel: [_ _ w8314] -> w8256
                                tunnel: w8254 -> [_ w8283 _]
                                frame #0 {
                                # "From here on 'True Volume being injected \nin this process' represents the true total \nvolume in this process"
                                n7806 = call "AbsolutePlungerPosition (SubVI).vi"("VISA Refnum in"=w8266) -> ("Plunger Position"=w8264:i32)  [unwired: 10 in]
                                n7807 = case shown="..\"Standard Pumping\"" w8265 {
                                tunnel: w8264 -> [w8274 w8282]
                                tunnel: w8263 -> [w8273 w8281]
                                tunnel: w8262 -> [w8270 w8278]
                                tunnel: [w8267 w8275] -> w8261
                                frame .."Standard Pumping" {
                                n7808 = Subtract(x=w8274, y=w8273) -> (x-y=w8272:dbl)
                                n7809 = Absolute Value(x=w8272) -> (abs(x)=w8271:dbl)
                                n7810 = Multiply(x=w8271, y=w8270) -> (x*y=w8269:dbl)
                                n7811 = Divide(x=w8269, y=3000.0) -> (x/y=w8267:dbl)
                                }
                                frame "High Resolution Pumping".. {
                                n7812 = Subtract(x=w8282, y=w8281) -> (x-y=w8280:dbl)
                                n7813 = Absolute Value(x=w8280) -> (abs(x)=w8279:dbl)
                                n7814 = Multiply(x=w8279, y=w8278) -> (x*y=w8277:dbl)
                                n7815 = Divide(x=w8277, y=24000.0) -> (x/y=w8275:dbl)
                                }
                                }
                                n7816 = local write "True Volume being \ninjected in this\nprocess"(w8261) -> ()
                                }
                                frame #1 {
                                # "From here on 'Volume being injected \nin this process' represents the volume \nin this sub process"
                                n7817 = call "AbsolutePlungerPosition (SubVI).vi"("VISA Refnum in"=w8288) -> ("Plunger Position"=w8286:i32)  [unwired: 10 in]
                                n7818 = case shown="..\"Standard Pumping\"" w8287 {
                                tunnel: w8286 -> [w8296 w8304]
                                tunnel: w8283 -> [w8295 w8303]
                                tunnel: w8285 -> [w8292 w8300]
                                tunnel: [w8289 w8297] -> w8284
                                frame .."Standard Pumping" {
                                n7819 = Subtract(x=w8296, y=w8295) -> (x-y=w8294:dbl)
                                n7820 = Absolute Value(x=w8294) -> (abs(x)=w8293:dbl)
                                n7821 = Multiply(x=w8293, y=w8292) -> (x*y=w8291:dbl)
                                n7822 = Divide(x=w8291, y=3000.0) -> (x/y=w8289:dbl)
                                }
                                frame "High Resolution Pumping".. {
                                n7823 = Subtract(x=w8304, y=w8303) -> (x-y=w8302:dbl)
                                n7824 = Absolute Value(x=w8302) -> (abs(x)=w8301:dbl)
                                n7825 = Multiply(x=w8301, y=w8300) -> (x*y=w8299:dbl)
                                n7826 = Divide(x=w8299, y=24000.0) -> (x/y=w8297:dbl)
                                }
                                }
                                n7827 = local write "Volume being Injected \nin this process"(w8284) -> ()
                                }
                                frame #2 {
                                n7828 = local read "Discard Volume"() -> (w8308:dbl)
                                n7829 = local read "Discard fluid \nprior to 1st \ndeposition"() -> (w8313:bool)
                                n7830 = local read "Volume being Injected \nin this process"() -> (w8312:dbl)
                                n7831 = Greater Or Equal?(x=w8312, y=w8308) -> (x >= y?=w8310:bool)
                                n7832 = call "AbsolutePlungerPositionStatus (SubVI).vi"("VISA Refnum in"=w8320) -> ("read buffer"=w8319:string)  [unwired: 10 in]
